vi "Treatment of NaN and Inf.vi"(7 "Treatment of Infinity/NaN":T1, 11 "Numeric Text":string) -> (3 "<JSON>":string)   [LabVIEW 2013, in "JSONtext support.lvlib"]
uses:
  JSONtext support.lvlib
  Infinity&NaN.ctl
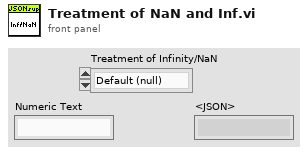
[diagram p1: front panel]
types:
  T1 = typedef "JSONtext support.lvlib/Infinity&NaN.ctl" = enum16{"Default (null)", "Extended", "LabVIEW extensions"}
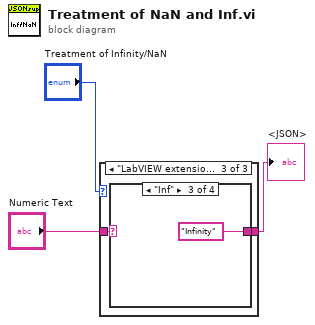
[diagram p0: block diagram]
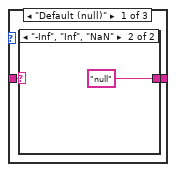
[diagram p2: hidden frame]
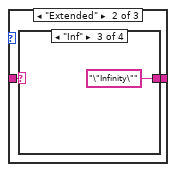
[diagram p4: hidden frame]
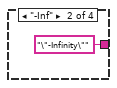
[diagram p6: hidden frame]
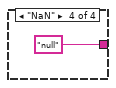
[diagram p7: hidden frame]
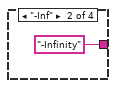
[diagram p9: hidden frame]
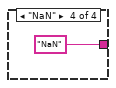
[diagram p10: hidden frame]
diagram:
  n1 = case shown="\"LabVIEW extensions\"" "Treatment of Infinity/NaN" {
    tunnel: "Numeric Text" -> [w5 w9 w15]
    tunnel: [w4 w8 w14] -> w2
    frame "Default (null)" {
      n2 = case shown="\"-Inf\", \"Inf\", \"NaN\"" w5 {
        selector: w5 -> [w6 _]
        tunnel: [w6 "null"] -> w4
        frame Default {
        }
        frame "-Inf", "Inf", "NaN" {
        }
      }
    }
    frame "Extended" {
      n3 = case shown="\"Inf\"" w9 {
        selector: w9 -> [w10 _ _ _]
        tunnel: [w10 "\"-Infinity\"" "\"Infinity\"" "null"] -> w8
        frame Default {
        }
        frame "-Inf" {
        }
        frame "Inf" {
        }
        frame "NaN" {
        }
      }
    }
    frame "LabVIEW extensions" {
      n4 = case shown="\"Inf\"" w15 {
        selector: w15 -> [w16 _ _ _]
        tunnel: [w16 "-Infinity" "Infinity" "NaN"] -> w14
        frame Default {
        }
        frame "-Inf" {
        }
        frame "Inf" {
        }
        frame "NaN" {
        }
      }
    }
  }
  "<JSON>" <- w2
